vi "P9P14_Temp_check_queue.vi"(8 "error in (no error)":errorcluster, 11 "Queue":refnum<queue> caption="5T Queue") -> (0 "error out":errorcluster, 1 "P9-P14 T-Cluster -Control":T1 {"Approach" items=["Fast Settle", "No O'Shoot"]}, 3 "New Entries?":bool)   [LabVIEW 2019]
uses:
  PPMS/P9P14-TCluster-Control.ctl
panel:
  out "Numeric":i32
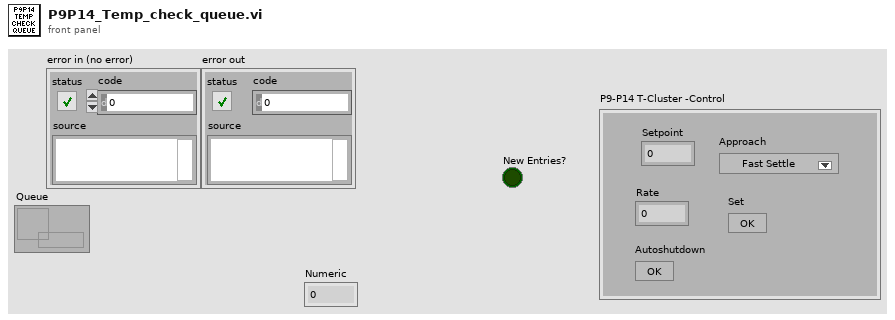
[diagram p1: front panel]
types:
  T1 = typedef "P9P14-TCluster-Control.ctl" = cluster{"Setpoint":dbl, "Rate":dbl, "Approach":u16, "Set":bool, "Autoshutdown":bool}
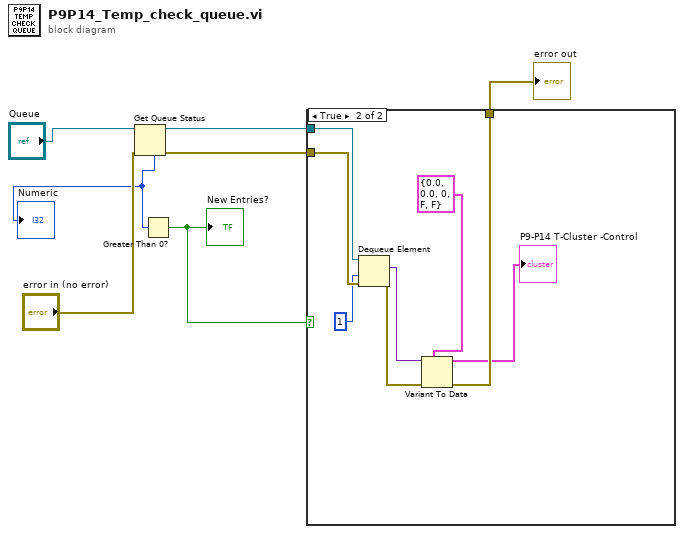
[diagram p0: block diagram]
diagram:
  n1 = Get Queue Status(queue="Queue", error in (no error)="error in (no error)") -> (queue out=w3:refnum<queue>, error out=w2:errorcluster, # elements in queue=w5:i32)  [unwired: 1 in, 5 out]
  "Numeric" <- w5
  n2 = Greater Than 0?(x=w5) -> (x > 0?=w4:bool)
  "New Entries?" <- w4
  n3 = case shown="True" w4 {
    tunnel: w3 -> [_ w16]
    tunnel: w2 -> [w8 w15]
    tunnel: [w8 w10] -> w1
    frame False {
    }
    frame True {
      n4 = Dequeue Element(queue=w16, timeout in ms (-1)=1, error in (no error)=w15) -> (element=w13:variant, error out=w12:errorcluster)  [unwired: 2 out]
      n5 = Variant To Data(error in=w12, type=T1 {"Setpoint"=0.0, "Rate"=0.0, "Approach"=0, "Set"=FALSE, "Autoshutdown"=FALSE} ("P9-P14 T-Cluster -Control"), Variant=w13) -> (data=→"P9-P14 T-Cluster -Control":T1, error out=w10:errorcluster)
    }
  }
  "error out" <- w1
